vi "SetParameter.vi"(8 "error in (no error)":errorcluster, 10 "SetParameter":T1, 11 "ChromaAcLoad in":refnum<class "ChromaAcLoad.lvclass">) -> (0 "error out":errorcluster, 2 "StatusUpdates":string[](array[string]), 3 "ChromaAcLoad out":refnum<class "ChromaAcLoad.lvclass">)   [LabVIEW 2018, in "AcPwrPlugins.lvlib" / "ChromaAcLoad.lvclass"]
uses:
  ChromaAcLoad.lvclass
  AcPwrBaseClass/TypeDefs/SetParameterInputs.ctl
  AcPwrBaseClass/AcPwrBase.lvclass
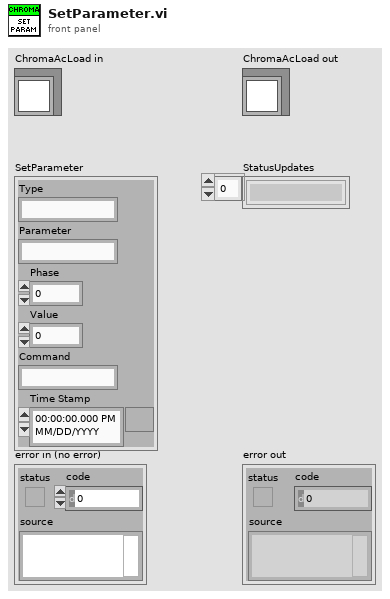
[diagram p1: front panel]
types:
  T1 = typedef "AcPwrPlugins.lvlib/AcPwrBase.lvclass/SetParameterInputs.ctl" = cluster{"Type":string, "Parameter":string, "Phase":i32, "Value":dbl, "Command":string, "Time Stamp":timestamp}
  T2 = typedef "AcPwrPlugins.lvlib/ChromaAcLoad.lvclass/Device(s)Settings.ctl" = cluster{"Configuration Mode":T3, "Phases":cluster{"Handle":string, "Name":string, "Phase Select":i32, "Instrument Options":string, "id query (T)":bool, "reset device (T)":bool, "Load Short Circuited":bool, "Line Synchronization":bool, "Load Current (A/Arms)":dbl, "Load Voltage (V/Vrms)":dbl, "Load Power (W)":dbl, "Load Resistance (Ohms)":dbl, "Load Current Peak Limit (A)":dbl, "Load Current Limit (A/Arms)":dbl, "Load Power Limit (W)":dbl, "Synch Frequency (Hz)":dbl, "Priority":enum16{"CF Only", "PF Only", "Both (CF)", "Both (PF)"}, "Crest Factor":dbl, "Power Factor":dbl, "Slew Rate":cluster{"Rise Slew Rate (A/ms)":i32, "Fall Slew Rate (A/ms)":i32}, "LC/RLC Mode":cluster{"Capacitance (uF)":i32, "Inductance (uH)":i32, "Series Resistance (Ohm)":dbl, "Parallel Resistance (Ohm)":dbl}, "Timing":cluster{"TimingOn":enum16{""}, "Hours":u32, "Minutes":u32, "Seconds":dbl, "CutoffVoltage":dbl}, "Connected":bool}[], "MeasName":string}
  T3 = typedef "ConfigMode.ctl" = enum16{"Constant Voltage (DC)", "Constant Power (DC)", "Constant Power (AC)", "Constant Current (DC)", "Constant Current (AC)", "Constant Resistance (DC)", "Constant Resistance (AC)", "Rectified Mode (DC)", "Inrush (AC)", "RLC CP (AC)", "RLC (AC)"}
  T4 = typedef "AcPwrPlugins.lvlib/ChromaAcLoad.lvclass/Measurements.ctl" = cluster{"Handle":string, "Name":string, "Enabled":bool, "Measurement Value":dbl, "Hold Peak Current Measurement":bool, "btnMeasFetch":bool, "ProtectionStatusString":string, "Measurement Type":T5}[]
  T5 = typedef "AcPwrPlugins.lvlib/ChromaAcLoad.lvclass/MeasurementType.ctl" = enum16{"Voltage (Vrms or V)", "Current (Arms or A)", "Power (W)", "Peak Voltage (V)", "Peak Current (A)", "Peak Power (W)", "Frequency (Hz)", "Resistance (Ohms)", "Voltage Overshoot (V)", "Positive Peak Current (A)", "Voltage Undershoot (V)", "Negative Peak Current (A)", "Apparent Power (VA)", "Reacitive Power (VAR)", "Voltage THD", "Power Factor", "Current's Crest Factor"}
  T6 = cluster{"Handle":string, "Name":string, "Phase Select":i32, "Instrument Options":string, "id query (T)":bool, "reset device (T)":bool, "Load Short Circuited":bool, "Line Synchronization":bool, "Load Current (A/Arms)":dbl, "Load Voltage (V/Vrms)":dbl, "Load Power (W)":dbl, "Load Resistance (Ohms)":dbl, "Load Current Peak Limit (A)":dbl, "Load Current Limit (A/Arms)":dbl, "Load Power Limit (W)":dbl, "Synch Frequency (Hz)":dbl, "Priority":enum16{"CF Only", "PF Only", "Both (CF)", "Both (PF)"}, "Crest Factor":dbl, "Power Factor":dbl, "Slew Rate":cluster{"Rise Slew Rate (A/ms)":i32, "Fall Slew Rate (A/ms)":i32}, "LC/RLC Mode":cluster{"Capacitance (uF)":i32, "Inductance (uH)":i32, "Series Resistance (Ohm)":dbl, "Parallel Resistance (Ohm)":dbl}, "Timing":cluster{"TimingOn":enum16{""}, "Hours":u32, "Minutes":u32, "Seconds":dbl, "CutoffVoltage":dbl}, "Connected":bool}[]
  T7 = cluster{"Handle":string, "Name":string, "Phase Select":i32, "Instrument Options":string, "id query (T)":bool, "reset device (T)":bool, "Load Short Circuited":bool, "Line Synchronization":bool, "Load Current (A/Arms)":dbl, "Load Voltage (V/Vrms)":dbl, "Load Power (W)":dbl, "Load Resistance (Ohms)":dbl, "Load Current Peak Limit (A)":dbl, "Load Current Limit (A/Arms)":dbl, "Load Power Limit (W)":dbl, "Synch Frequency (Hz)":dbl, "Priority":enum16{"CF Only", "PF Only", "Both (CF)", "Both (PF)"}, "Crest Factor":dbl, "Power Factor":dbl, "Slew Rate":cluster{"Rise Slew Rate (A/ms)":i32, "Fall Slew Rate (A/ms)":i32}, "LC/RLC Mode":cluster{"Capacitance (uF)":i32, "Inductance (uH)":i32, "Series Resistance (Ohm)":dbl, "Parallel Resistance (Ohm)":dbl}, "Timing":cluster{"TimingOn":enum16{""}, "Hours":u32, "Minutes":u32, "Seconds":dbl, "CutoffVoltage":dbl}, "Connected":bool}
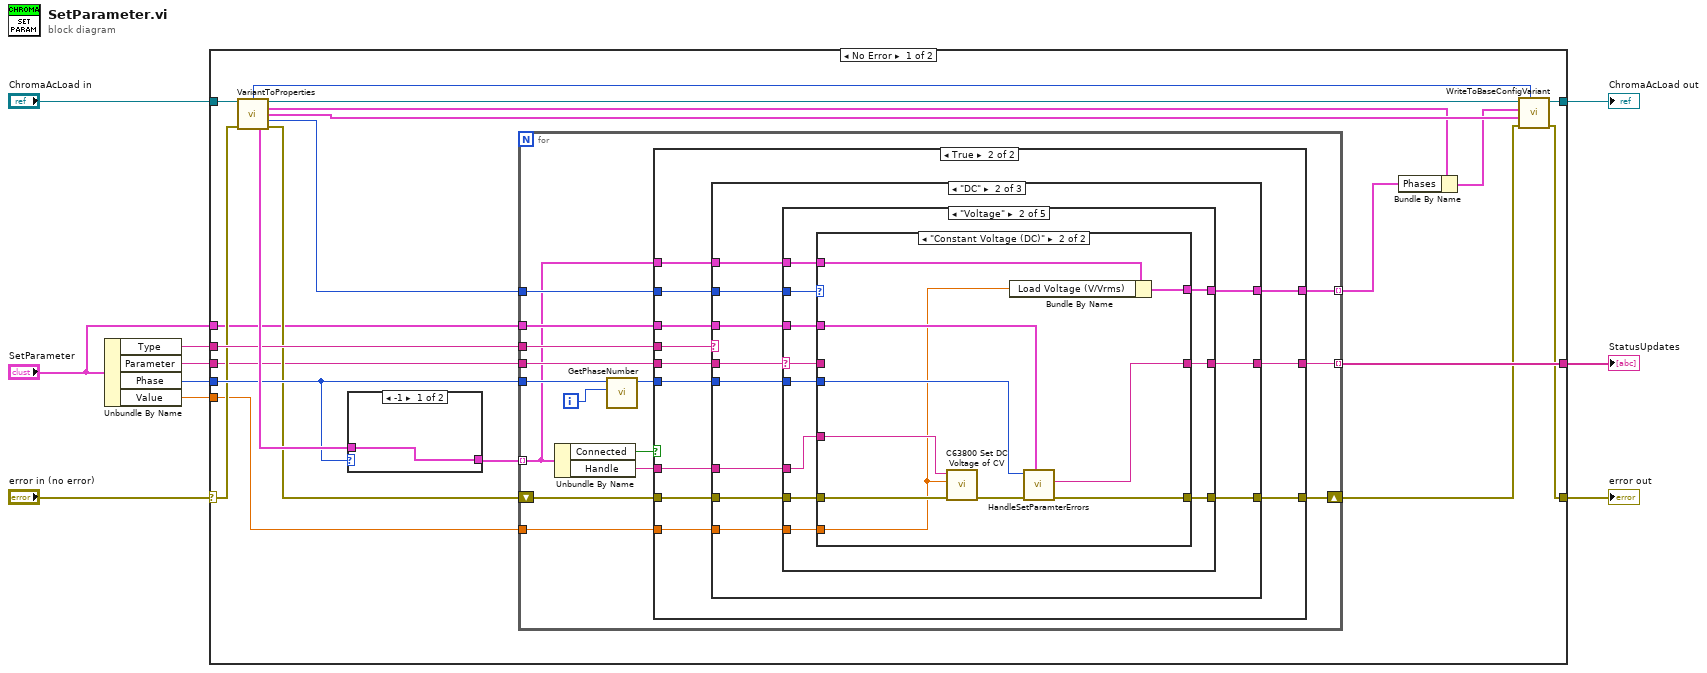
[diagram p0: block diagram]
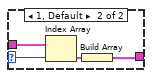
[diagram p2: hidden frame]
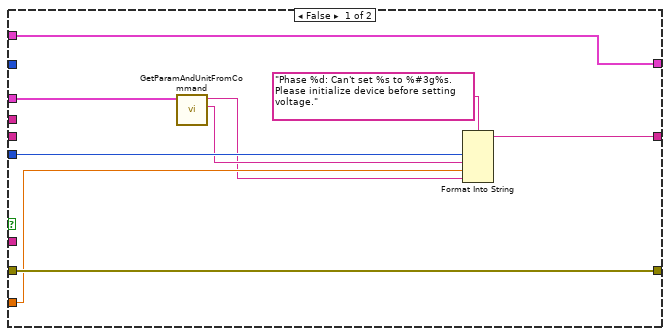
[diagram p3: hidden frame]
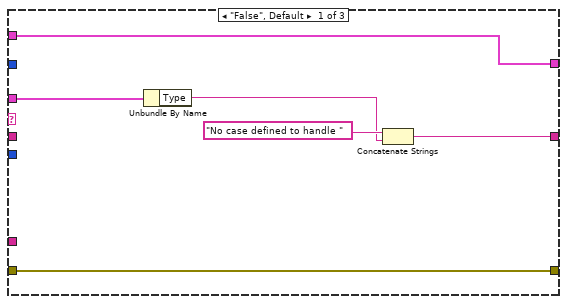
[diagram p4: hidden frame]
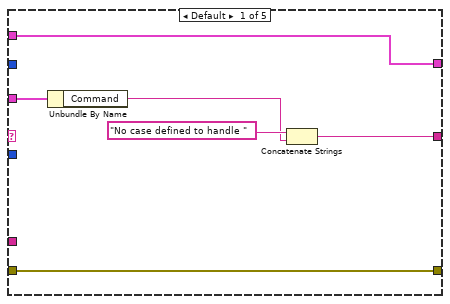
[diagram p5: hidden frame]
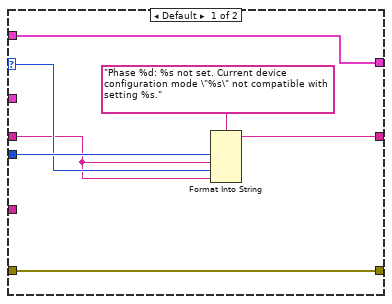
[diagram p6: hidden frame]
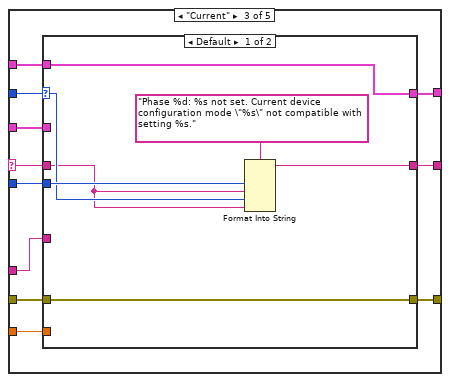
[diagram p7: hidden frame]
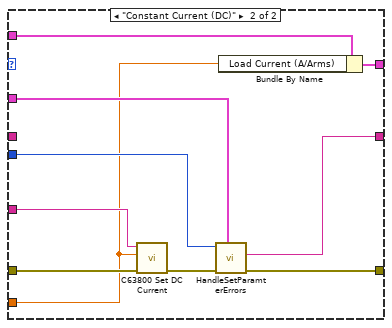
[diagram p8: hidden frame]
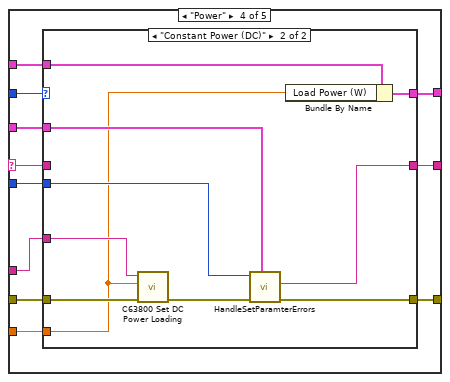
[diagram p9: hidden frame]
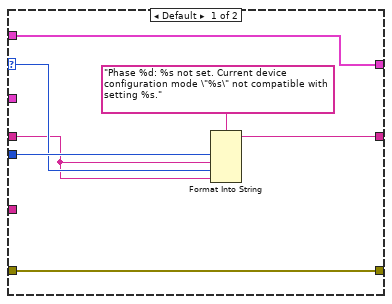
[diagram p10: hidden frame]
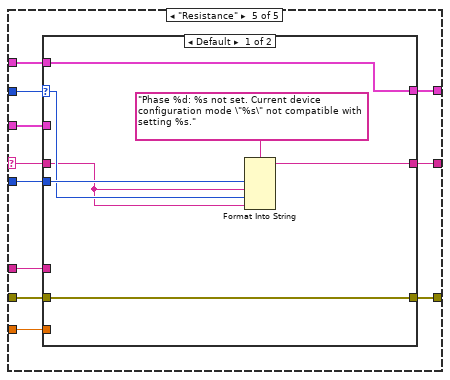
[diagram p11: hidden frame]
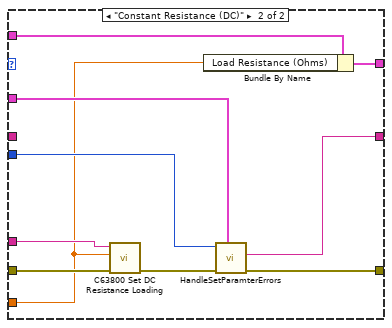
[diagram p12: hidden frame]
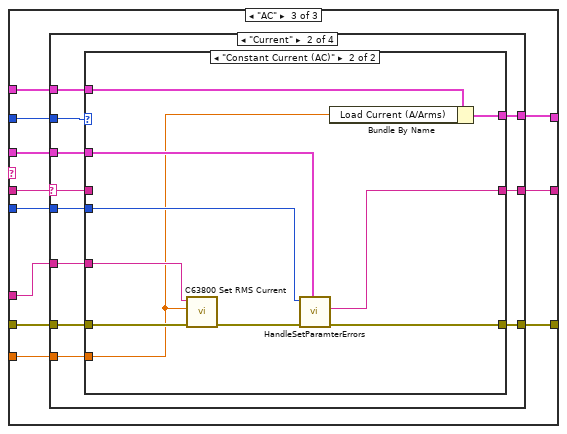
[diagram p13: hidden frame]
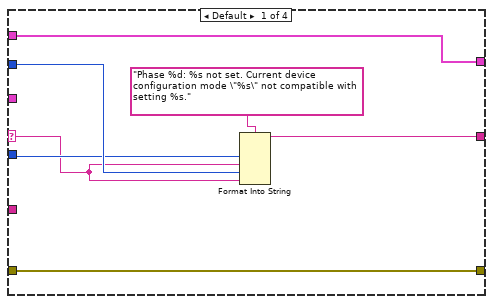
[diagram p14: hidden frame]
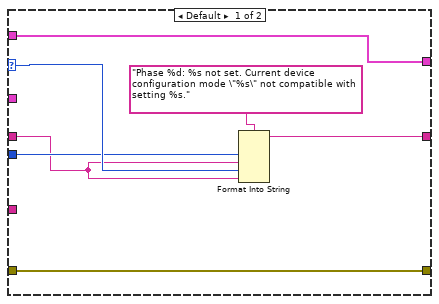
[diagram p15: hidden frame]
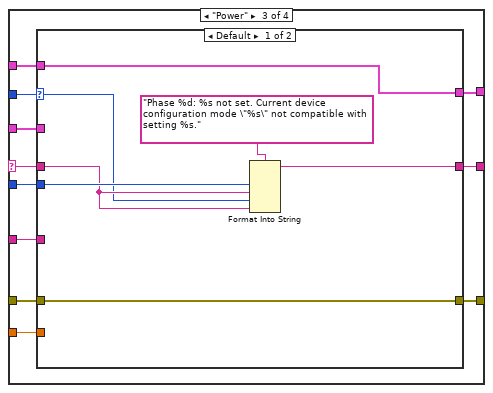
[diagram p16: hidden frame]
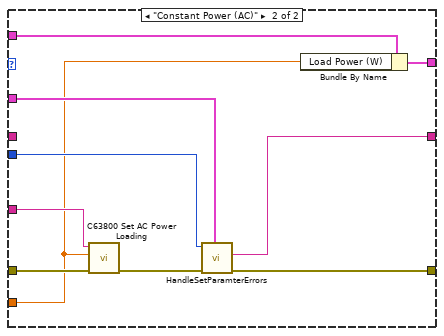
[diagram p17: hidden frame]
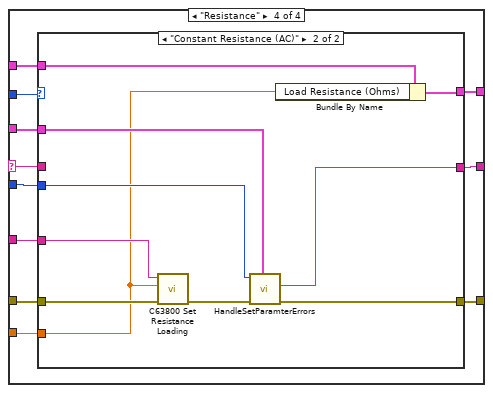
[diagram p18: hidden frame]
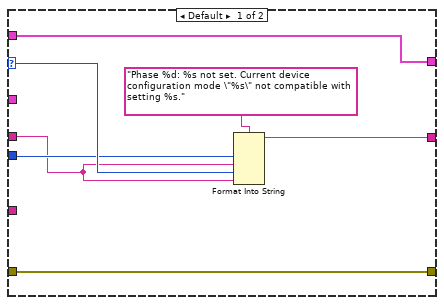
[diagram p19: hidden frame]
diagram:
  n1 = Unbundle By Name("SetParameter") -> ("Type"=w3:string, "Parameter"=w2:string, "Phase"=w5:i32, "Value"=w4:dbl)
  n2 = case shown="No Error" "error in (no error)" {
    selector: "error in (no error)" -> [w24 w311]
    tunnel: "ChromaAcLoad in" -> [w31 w310]
    tunnel: [w18 w310] -> w9
    tunnel: w5 -> [w27 _]
    tunnel: [w26 _] -> w8
    tunnel: w3 -> [w25 _]
    tunnel: [w15 w311] -> w6
    tunnel: w4 -> [w22 _]
    tunnel: w2 -> [w21 _]
    tunnel: "SetParameter" -> [w20 _]
    frame No Error {
      n3 = call "VariantToProperties.vi"("ChromaAcLoad"=w31, "error in (no error)"=w24) -> ("ChromaAcLoad"=w19:refnum<class "ChromaAcLoad.lvclass">, "Device Properties"=w14:T2, "Meas"=w17:T4, "Configuration Mode"=w28:T3, "Measurement Refresh Time (ms)"=w11:u32, "Phases"=w30:T6, "error out"=w23:errorcluster)  [unwired: 7 in]
      n4 = case shown="-1" w27 {
        selector: w27 -> [_ w33]
        tunnel: w30 -> [w32 w36]
        tunnel: [w32 w34] -> w29
        frame -1 {
        }
        frame 1, Default {
          n5 = Index Array(array=w36, index=w33) -> (element=w35:T7)
          n6 = Build Array(w35) -> (w34:T6)
        }
      }
      n7 = for {
        tunnel: w29 -> [w38] mode=indexing
        shift-right: [w50] -> w16
        shift-left: w23 -> [w51]
        tunnel: w22 -> [w47]
        tunnel: w28 -> [w46]
        tunnel: w27 -> [w44]
        tunnel: [w42] -> w26 mode=indexing
        tunnel: w25 -> [w41]
        tunnel: w21 -> [w40]
        tunnel: w20 -> [w39]
        tunnel: [w37] -> w13 mode=indexing
        i -> [w45]
        n8 = Unbundle By Name(w38) -> ("Connected"=w49:bool, "Handle"=w48:string)
        n9 = call "GetPhaseNumber.vi"("Loop Counter"=w45, "Phase(-1, all) in"=w44) -> ("Phase(-1, all) out"=w43:i32)  [unwired: 9 in]
        n10 = case shown="True" w49 {
          tunnel: w51 -> [w60 w72]
          tunnel: [w60 w71] -> w50
          tunnel: w48 -> [_ w70]
          tunnel: w47 -> [w54 w69]
          tunnel: w46 -> [_ w68]
          tunnel: w43 -> [w59 w67]
          tunnel: [w57 w66] -> w42
          tunnel: w41 -> [_ w65]
          tunnel: w40 -> [_ w64]
          tunnel: w39 -> [w56 w63]
          tunnel: w38 -> [w52 w62]
          tunnel: [w52 w61] -> w37
          frame False {
            n11 = call "GetParamAndUnitFromCommand.vi"("SetParameter"=w56) -> ("Parameter"=w55:string, "Unit Label"=w53:string)  [unwired: 9 in]
            n12 = Format Into String(format string="Phase %d: Can't set %s to %#3g%s. Please initialize device before setting voltage.", w59, w55, w54, w53) -> (resulting string=w57:string)  [unwired: 2 in, 1 out]
          }
          frame True {
            n13 = case shown="\"DC\"" w65 {
              tunnel: w72 -> [w74 w89 w216]
              tunnel: [w74 w88 w215] -> w71
              tunnel: w70 -> [_ w87 w214]
              tunnel: w69 -> [_ w86 w213]
              tunnel: w68 -> [_ w85 w217]
              tunnel: w67 -> [_ w84 w211]
              tunnel: [w75 w83 w210] -> w66
              tunnel: w64 -> [_ w82 w218]
              tunnel: w63 -> [w76 w81 w212]
              tunnel: w62 -> [w73 w80 w209]
              tunnel: [w73 w79 w208] -> w61
              frame "False", Default {
                n14 = Unbundle By Name(w76) -> ("Type"=w77:string)
                n15 = Concatenate Strings("No case defined to handle " ("string"), w77) -> (w75:string)
              }
              frame "DC" {
                n16 = case shown="\"Voltage\"" w82 {
                  selector: w82 -> [_ w99 w126 w154 w182]
                  tunnel: w89 -> [w95 w106 w134 w162 w190]
                  tunnel: [w95 w105 w133 w161 w189] -> w88
                  tunnel: w87 -> [_ w104 w132 w160 w188]
                  tunnel: w86 -> [_ w103 w131 w159 w187]
                  tunnel: w85 -> [_ w102 w130 w158 w186]
                  tunnel: w84 -> [_ w101 w129 w157 w185]
                  tunnel: [w94 w100 w128 w156 w184] -> w83
                  tunnel: w81 -> [w92 w98 w127 w155 w183]
                  tunnel: w80 -> [w90 w97 w125 w153 w181]
                  tunnel: [w90 w96 w124 w152 w180] -> w79
                  frame Default {
                    n17 = Unbundle By Name(w92) -> ("Command"=w91:string)
                    n18 = Concatenate Strings("No case defined to handle " ("string"), w91) -> (w94:string)
                  }
                  frame "Voltage" {
                    n19 = case shown="\"Constant Voltage (DC)\"" w102 {
                      selector: w102 -> [w109 _]
                      tunnel: w106 -> [w113 w123]
                      tunnel: [w113 w120] -> w105
                      tunnel: w104 -> [_ w122]
                      tunnel: w103 -> [_ w115]
                      tunnel: w101 -> [w111 w119]
                      tunnel: [w110 w118] -> w100
                      tunnel: w98 -> [_ w117]
                      tunnel: w99 -> [w108 _]
                      tunnel: w97 -> [w107 w116]
                      tunnel: [w107 w114] -> w96
                      frame Default {
                        n20 = Format Into String(format string="Phase %d: %s not set. Current device configuration mode \"%s\" not compatible with setting %s.", w111, w108, w109, w108) -> (resulting string=w110:string)  [unwired: 2 in, 1 out]
                      }
                      frame "Constant Voltage (DC)" {
                        n21 = call <instrlib>:"C63800 Set DC Voltage of CV.vi"("error in (no error)"=w123, "SetDCVoltageofCV"=w115, "Instrument Handle"=w122) -> ("error out"=w121:errorcluster)  [unwired: 7 in, 1 out]
                        n22 = Bundle By Name(cluster=w116, "Load Voltage (V/Vrms)"=w115) -> (w114:T7)
                        n23 = call "HandleSetParamterErrors.vi"("SetParameter"=w117, "error in (no error)"=w121, "Phase"=w119) -> ("error IO"=w120:errorcluster, "Status Update"=w118:string)  [unwired: 7 in]
                      }
                    }
                  }
                  frame "Current" {
                    n24 = case shown="Default" w130 {
                      selector: w130 -> [w137 _]
                      tunnel: w134 -> [w141 w146]
                      tunnel: [w141 w151] -> w133
                      tunnel: w132 -> [_ w147]
                      tunnel: w131 -> [_ w143]
                      tunnel: w129 -> [w139 w150]
                      tunnel: [w138 w149] -> w128
                      tunnel: w127 -> [_ w148]
                      tunnel: w126 -> [w136 _]
                      tunnel: w125 -> [w135 w144]
                      tunnel: [w135 w142] -> w124
                      frame Default {
                        n25 = Format Into String(format string="Phase %d: %s not set. Current device configuration mode \"%s\" not compatible with setting %s.", w139, w136, w137, w136) -> (resulting string=w138:string)  [unwired: 2 in, 1 out]
                      }
                      frame "Constant Current (DC)" {
                        n26 = call <instrlib>:"C63800 Set DC Current.vi"("error in (no error)"=w146, "Set DC Current"=w143, "Instrument Handle"=w147) -> ("error out"=w145:errorcluster)  [unwired: 7 in, 1 out]
                        n27 = call "HandleSetParamterErrors.vi"("SetParameter"=w148, "error in (no error)"=w145, "Phase"=w150) -> ("error IO"=w151:errorcluster, "Status Update"=w149:string)  [unwired: 7 in]
                        n28 = Bundle By Name(cluster=w144, "Load Current (A/Arms)"=w143) -> (w142:T7)
                      }
                    }
                  }
                  frame "Power" {
                    n29 = case shown="\"Constant Power (DC)\"" w158 {
                      selector: w158 -> [w165 _]
                      tunnel: w162 -> [w169 w175]
                      tunnel: [w169 w179] -> w161
                      tunnel: w160 -> [_ w173]
                      tunnel: w159 -> [_ w170]
                      tunnel: w157 -> [w167 w178]
                      tunnel: [w166 w177] -> w156
                      tunnel: w155 -> [_ w176]
                      tunnel: w154 -> [w164 _]
                      tunnel: w153 -> [w163 w172]
                      tunnel: [w163 w171] -> w152
                      frame Default {
                        n30 = Format Into String(format string="Phase %d: %s not set. Current device configuration mode \"%s\" not compatible with setting %s.", w167, w164, w165, w164) -> (resulting string=w166:string)  [unwired: 2 in, 1 out]
                      }
                      frame "Constant Power (DC)" {
                        n31 = call <instrlib>:"C63800 Set DC Power Loading.vi"("error in (no error)"=w175, "DC Power Loading"=w170, "Instrument Handle"=w173) -> ("error out"=w174:errorcluster)  [unwired: 7 in, 1 out]
                        n32 = call "HandleSetParamterErrors.vi"("SetParameter"=w176, "error in (no error)"=w174, "Phase"=w178) -> ("error IO"=w179:errorcluster, "Status Update"=w177:string)  [unwired: 7 in]
                        n33 = Bundle By Name(cluster=w172, "Load Power (W)"=w170) -> (w171:T7)
                      }
                    }
                  }
                  frame "Resistance" {
                    n34 = case shown="Default" w186 {
                      selector: w186 -> [w193 _]
                      tunnel: w190 -> [w197 w203]
                      tunnel: [w197 w207] -> w189
                      tunnel: w188 -> [_ w201]
                      tunnel: w187 -> [_ w199]
                      tunnel: w185 -> [w195 w206]
                      tunnel: [w194 w205] -> w184
                      tunnel: w183 -> [_ w204]
                      tunnel: w182 -> [w192 _]
                      tunnel: w181 -> [w191 w200]
                      tunnel: [w191 w198] -> w180
                      frame Default {
                        n35 = Format Into String(format string="Phase %d: %s not set. Current device configuration mode \"%s\" not compatible with setting %s.", w195, w192, w193, w192) -> (resulting string=w194:string)  [unwired: 2 in, 1 out]
                      }
                      frame "Constant Resistance (DC)" {
                        n36 = call <instrlib>:"C63800 Set DC Resistance Loading.vi"("error in (no error)"=w203, "DC Resistance Loading"=w199, "Instrument Handle"=w201) -> ("error out"=w202:errorcluster)  [unwired: 7 in, 1 out]
                        n37 = Bundle By Name(cluster=w200, "Load Resistance (Ohms)"=w199) -> (w198:T7)
                        n38 = call "HandleSetParamterErrors.vi"("SetParameter"=w204, "error in (no error)"=w202, "Phase"=w206) -> ("error IO"=w207:errorcluster, "Status Update"=w205:string)  [unwired: 7 in]
                      }
                    }
                  }
                }
              }
              frame "AC" {
                n39 = case shown="\"Current\"" w218 {
                  selector: w218 -> [w220 w228 w256 w285]
                  tunnel: w217 -> [w222 w236 w264 w292]
                  tunnel: w216 -> [w225 w234 w263 w290]
                  tunnel: [w225 w230 w262 w284] -> w215
                  tunnel: w214 -> [_ w235 w261 w291]
                  tunnel: w213 -> [_ w233 w260 w289]
                  tunnel: w212 -> [_ w231 w259 w288]
                  tunnel: w211 -> [w221 w232 w258 w287]
                  tunnel: [w223 w229 w257 w286] -> w210
                  tunnel: w209 -> [w219 w227 w255 w282]
                  tunnel: [w219 w226 w254 w283] -> w208
                  frame Default {
                    n40 = Format Into String(format string="Phase %d: %s not set. Current device configuration mode \"%s\" not compatible with setting %s.", w221, w220, w222, w220) -> (resulting string=w223:string)  [unwired: 2 in, 1 out]
                  }
                  frame "Current" {
                    n41 = case shown="\"Constant Current (AC)\"" w236 {
                      selector: w236 -> [w242 _]
                      tunnel: w235 -> [_ w252]
                      tunnel: w234 -> [w238 w251]
                      tunnel: w233 -> [_ w244]
                      tunnel: w232 -> [w241 w250]
                      tunnel: w231 -> [_ w249]
                      tunnel: [w238 w248] -> w230
                      tunnel: [w240 w247] -> w229
                      tunnel: w228 -> [w239 _]
                      tunnel: w227 -> [w237 w246]
                      tunnel: [w237 w245] -> w226
                      frame Default {
                        n42 = Format Into String(format string="Phase %d: %s not set. Current device configuration mode \"%s\" not compatible with setting %s.", w241, w239, w242, w239) -> (resulting string=w240:string)  [unwired: 2 in, 1 out]
                      }
                      frame "Constant Current (AC)" {
                        n43 = call <instrlib>:"C63800 Set RMS Current.vi"("error in (no error)"=w251, "Set RMS Current"=w244, "Instrument Handle"=w252) -> ("error out"=w253:errorcluster)  [unwired: 7 in, 1 out]
                        n44 = call "HandleSetParamterErrors.vi"("SetParameter"=w249, "error in (no error)"=w253, "Phase"=w250) -> ("error IO"=w248:errorcluster, "Status Update"=w247:string)  [unwired: 7 in]
                        n45 = Bundle By Name(cluster=w246, "Load Current (A/Arms)"=w244) -> (w245:T7)
                      }
                    }
                  }
                  frame "Power" {
                    n46 = case shown="Default" w264 {
                      selector: w264 -> [w267 _]
                      tunnel: w263 -> [w271 w281]
                      tunnel: [w271 w279] -> w262
                      tunnel: w261 -> [_ w278]
                      tunnel: w260 -> [_ w273]
                      tunnel: w259 -> [_ w277]
                      tunnel: w258 -> [w269 w276]
                      tunnel: [w266 w275] -> w257
                      tunnel: w256 -> [w268 _]
                      tunnel: w255 -> [w265 w274]
                      tunnel: [w265 w272] -> w254
                      frame Default {
                        n47 = Format Into String(format string="Phase %d: %s not set. Current device configuration mode \"%s\" not compatible with setting %s.", w269, w268, w267, w268) -> (resulting string=w266:string)  [unwired: 2 in, 1 out]
                      }
                      frame "Constant Power (AC)" {
                        n48 = call <instrlib>:"C63800 Set AC Power Loading.vi"("error in (no error)"=w281, "AC Power Loading"=w273, "Instrument Handle"=w278) -> ("error out"=w280:errorcluster)  [unwired: 7 in, 1 out]
                        n49 = call "HandleSetParamterErrors.vi"("SetParameter"=w277, "error in (no error)"=w280, "Phase"=w276) -> ("error IO"=w279:errorcluster, "Status Update"=w275:string)  [unwired: 7 in]
                        n50 = Bundle By Name(cluster=w274, "Load Power (W)"=w273) -> (w272:T7)
                      }
                    }
                  }
                  frame "Resistance" {
                    n51 = case shown="\"Constant Resistance (AC)\"" w292 {
                      selector: w292 -> [w297 _]
                      tunnel: w291 -> [_ w308]
                      tunnel: w290 -> [w294 w307]
                      tunnel: w289 -> [_ w300]
                      tunnel: w288 -> [_ w306]
                      tunnel: w287 -> [w296 w305]
                      tunnel: [w298 w304] -> w286
                      tunnel: w285 -> [w295 _]
                      tunnel: [w294 w303] -> w284
                      tunnel: [w293 w301] -> w283
                      tunnel: w282 -> [w293 w302]
                      frame Default {
                        n52 = Format Into String(format string="Phase %d: %s not set. Current device configuration mode \"%s\" not compatible with setting %s.", w296, w295, w297, w295) -> (resulting string=w298:string)  [unwired: 2 in, 1 out]
                      }
                      frame "Constant Resistance (AC)" {
                        n53 = call <instrlib>:"C63800 Set Resistance Loading.vi"("error in (no error)"=w307, "Resistance Loading"=w300, "Instrument Handle"=w308) -> ("error out"=w309:errorcluster)  [unwired: 7 in, 1 out]
                        n54 = call "HandleSetParamterErrors.vi"("SetParameter"=w306, "error in (no error)"=w309, "Phase"=w305) -> ("error IO"=w303:errorcluster, "Status Update"=w304:string)  [unwired: 7 in]
                        n55 = Bundle By Name(cluster=w302, "Load Resistance (Ohms)"=w300) -> (w301:T7)
                      }
                    }
                  }
                }
              }
            }
          }
        }
      }
      n56 = Bundle By Name(cluster=w14, "Phases"=w13) -> (w12:T2)
      n57 = call "WriteToBaseConfigVariant.vi"("Measurement Refresh Time (ms)"=w11, "error in (no error)"=w16, "Meas"=w17, "Config"=w12, "ChromaAcLoad in"=w19) -> ("error out"=w15:errorcluster, "ChromaAcLoad out"=w18:refnum<class "ChromaAcLoad.lvclass">)  [unwired: 5 in]
    }
    frame Error {
    }
  }
  "error out" <- w6
  "ChromaAcLoad out" <- w9
  "StatusUpdates" <- w8
